vi "Detect Falling Edge (SubVI).vi"(2 "Trigger":bool) -> (0 "8-bit Count (0-63)":u8)   [LabVIEW 2015]
doc: "This VI supports a falling edge event counter. When the input trigger creates a falling edge, the value of 8-bit Count is incremented on the host VI."
panel:
  # "This VI supports a falling edge event counter.  When the input trigger creates a falling edge, the value of 8-bit Count is incremented on the host VI."
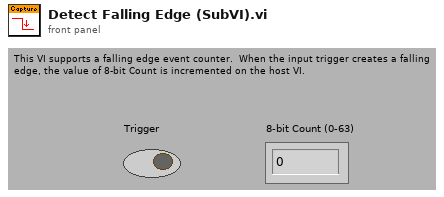
[diagram p1: front panel]
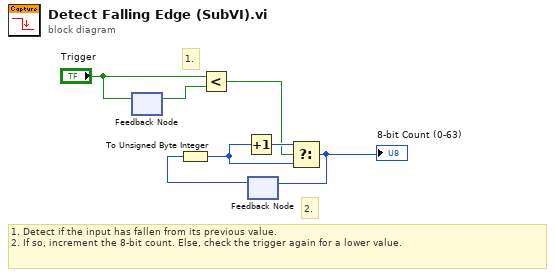
[diagram p0: block diagram]
diagram:
  # "1."
  # "2."
  # "1. Detect if the input has fallen from its previous value.\n2. If so, increment the 8-bit count. Else, check the trigger again for a lower value."
  n1 = feedback-in #1("Trigger") -> ()
  n2 = feedback #1() -> (w5:bool)  [unwired: 1 out]
  n3 = Less?(x="Trigger", y=w5) -> (x < y?=w6:bool)
  n4 = feedback #2() -> (w2:u8)  [unwired: 1 out]
  n5 = To Unsigned Byte Integer(number=w2) -> (unsigned 8bit integer=w1:u8)
  n6 = Increment(x=w1) -> (x+1=w7:u8)
  n7 = Select(t=w7, s=w6, f=w1) -> (s? t:f=w4:u8)
  "8-bit Count (0-63)" <- w4
  n8 = feedback-in #2(w4) -> ()
